vi "EnableDisable.vi"(1 "EN?":bool) -> (0 "Mode":T1(ring))   [LabVIEW 2024]
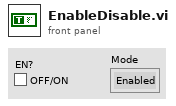
[diagram p1: front panel]
types:
  T1 = enum8{"Enabled", "Disabled", "Disabled and Grayed Out"}
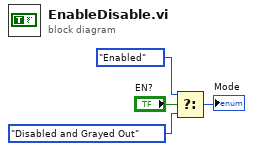
[diagram p0: block diagram]
diagram:
  n1 = Select(t=T1."Enabled" ("Disabled"), s="EN?", f=T1."Disabled and Grayed Out" ("Disabled")) -> (s? t:f=→"Mode":T1)
